vi "Page_Info_Validate_Filename.vi"(8 "error in (no error)":errorcluster, 10 "Filename in":string, 11 "AB_DLL in":refnum<class "AB_DLL.lvclass">) -> (0 "error out":errorcluster, 1 "hasInvalidCharacters":bool, 2 "Filename out":string, 3 "AB_DLL out":refnum<class "AB_DLL.lvclass">, 5 "message":string)   [LabVIEW 2020, in "AB_DLL.lvclass"]
uses:
  <vilib>/AppBuilder/AB_Classes/DLL/AB_DLL.lvclass
  e:/builds/penguin/labview/branches/2020/dev/dist/vi.lib/AppBuilder/AB_Classes/Build/AB_Build.lvclass
  <vilib>/AppBuilder/AB_Classes/Application/AB_Application.lvclass
  <vilib>/AppBuilder/AB_Classes/Build/AB_Build.lvclass
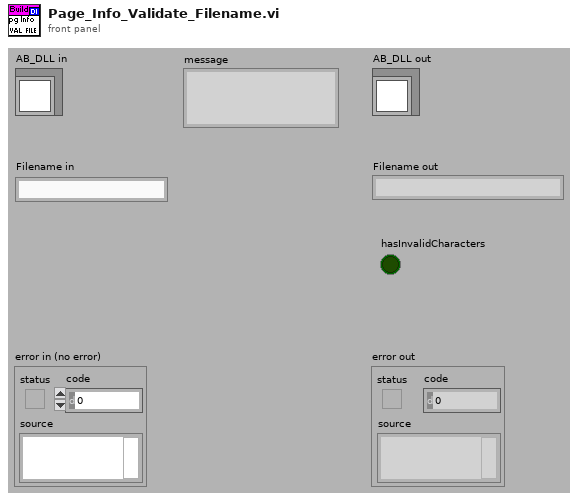
[diagram p1: front panel]
types:
  T1 = enum32{"invalid OS target", "Mac OS", "Windows 3.1", "Windows 95/NT", "Solaris 1", "Solaris 2", "HP-UX", "PowerMAX", "Linux", "Irix", "Rhapsody", "BeOS", "AIX", "OSF1", "VxWorks", "PharLap", "Carbon", "RTX", "Windows x64", "Linux x64", "Mac OS X x64"}
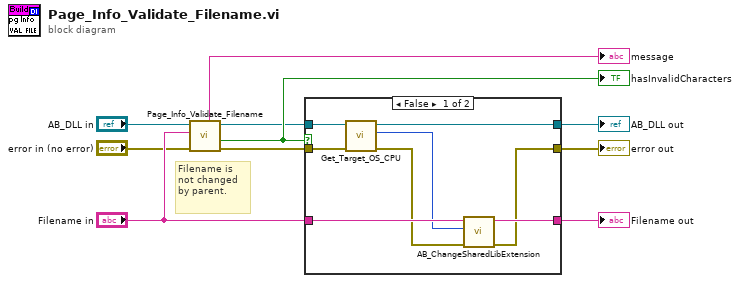
[diagram p0: block diagram]
diagram:
  # "Filename is not changed by parent."
  n1 = call-parent "Page_Info_Validate_Filename.vi"("error in (no error)"="error in (no error)", "Filename in"="Filename in", "AB_Targetfile in"="AB_DLL in") -> ("error out"=w3:errorcluster, "hasInvalidCharacters"=w7:bool, "AB_Targetfile out"=w5:refnum<class "AB_DLL.lvclass">, "message"=→"message":string)  [unwired: 4 in, 1 out]
  "hasInvalidCharacters" <- w7
  n2 = case shown="False" w7 {
    tunnel: [w18 w21] -> w8
    tunnel: "Filename in" -> [w17 w21]
    tunnel: w5 -> [w15 w20]
    tunnel: [w14 w20] -> w4
    tunnel: w3 -> [w12 w19]
    tunnel: [w16 w19] -> w1
    frame False {
      n3 = call <vilib>:"Get_Target_OS_CPU.vi"("error in (no error)"=w12, "AB_Build in"=w15) -> ("error out"=w13:errorcluster, "Target Operating System"=w11:T1, "AB_Build out"=w14:refnum<class "AB_DLL.lvclass">)  [unwired: 6 in, 1 out]
      n4 = call <vilib>:"AB_ChangeSharedLibExtension.vi"("error in (no error)"=w13, "Target OS"=w11, "Target file name"=w17) -> ("error out"=w16:errorcluster, "New target file name"=w18:string)  [unwired: 7 in]
    }
    frame True {
    }
  }
  "error out" <- w1
  "AB_DLL out" <- w4
  "Filename out" <- w8
